vi "GetFirstTagByKeyword.vi"(10 "keyword":string, 11 "tags":T1[](array[typedef])) -> (3 "first tag":T1)   [LabVIEW 2017, in "DeviceModelHelpers.lvlib"]
doc: "Returns the first tag associated with a specific keyword."
uses:
  <vilib>/addons/InsightCM/Utilities/DeviceModelHelpers/DeviceModelHelpers.lvlib
  <vilib>/addons/InsightCM/MessageBus/Base/controls/Tag.ctl
  <vilib>/addons/InsightCM/MessageBus/Base/controls/KeyValuePair.ctl
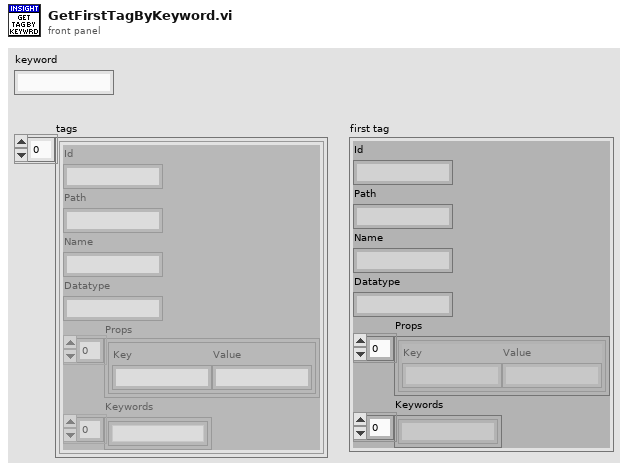
[diagram p1: front panel]
types:
  T1 = typedef "Tag.ctl" = cluster{"Id":string, "Path":string, "Name":string, "Datatype":string, "Props":T2[], "Keywords":string[]}
  T2 = typedef "KeyValuePair.ctl" = cluster{"Key":string, "Value":string}
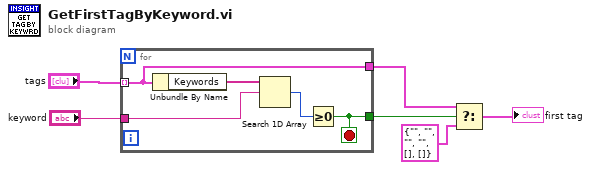
[diagram p0: block diagram]
diagram:
  n1 = for {
    tunnel: "tags" -> [w8] mode=indexing
    tunnel: "keyword" -> [w10]
    tunnel: [w8] -> w3
    tunnel: [w7] -> w4
    stop <- w7 stop-if-true
    n2 = Unbundle By Name(w8) -> ("Keywords"=w11:string[])
    n3 = Search 1D Array(1D array=w11, element=w10) -> (index of element=w9:i32)  [unwired: 1 in]
    n4 = Greater Or Equal To 0?(x=w9) -> (x >= 0?=w7:bool)
  }
  n5 = Select(t=w3, s=w4, f=T1 {"Id"="", "Path"="", "Name"="", "Datatype"="", "Props"=[], "Keywords"=[]}) -> (s? t:f=→"first tag":T1)
